vi "Message Log Exited MHLC.vi"(8 "error in (no error)":errorcluster, 10 "Data in":variant, 11 "Debug Server in":refnum<class "Debug Server.lvclass">) -> (0 "error out":errorcluster, 3 "Debug Server out":refnum<class "Debug Server.lvclass">)   [LabVIEW 2017, in "Debug Server.lvclass"]
doc: "A Message Log has exited. Remove it from the array of open Message Logs. Tell TCP Server that the Message Log no longer exists."
uses:
  Debug Server.lvclass
  C:/Program Files (x86)/National Instruments/LabVIEW 2017/vi.lib/addons/_Workers/Library/Classes/Worker/Worker.lvclass
  Debug Server.lvclass/Debug Server.ctl
  Debug Server TCP Server and Client/Workers/DS TCP Server/rqp_Message Log Exited.ctl
  Common VIs/DC_UID.ctl
  <vilib>/Utility/error.llb/Error Cluster From Error Code.vi
  <vilib>/ErrorRing/Error Ring.xnode
  Message Log/Message Log.lvclass
  Debug Server TCP Server and Client/Workers/DS TCP Server/DS TCP Server.lvclass
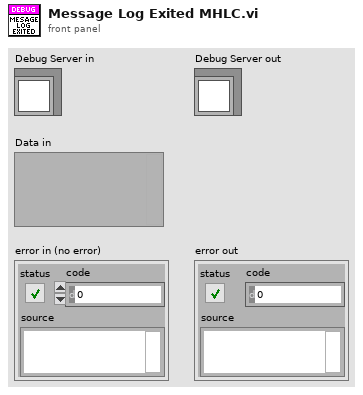
[diagram p1: front panel]
types:
  T1 = typedef "Message Log.lvclass/rsp_Message Log Exited.ctl" = cluster{"Message Log ID":T2}
  T2 = typedef "Message Log ID.ctl" = cluster{"Head Worker ID":string, "IP Address":string}
  T3 = typedef "Debug Server.lvclass/Dynamic Message Log Data.ctl" = cluster{"Message Log":refnum<class "Message Log.lvclass">, "DC_UID":T4, "Message Log ID":T2}
  T4 = typedef "DC_UID.ctl" = string
  T5 = typedef "DS TCP Server.lvlib/DS TCP Server.lvclass/rqp_Message Log Exited.ctl" = cluster{"DC_UID":T4}
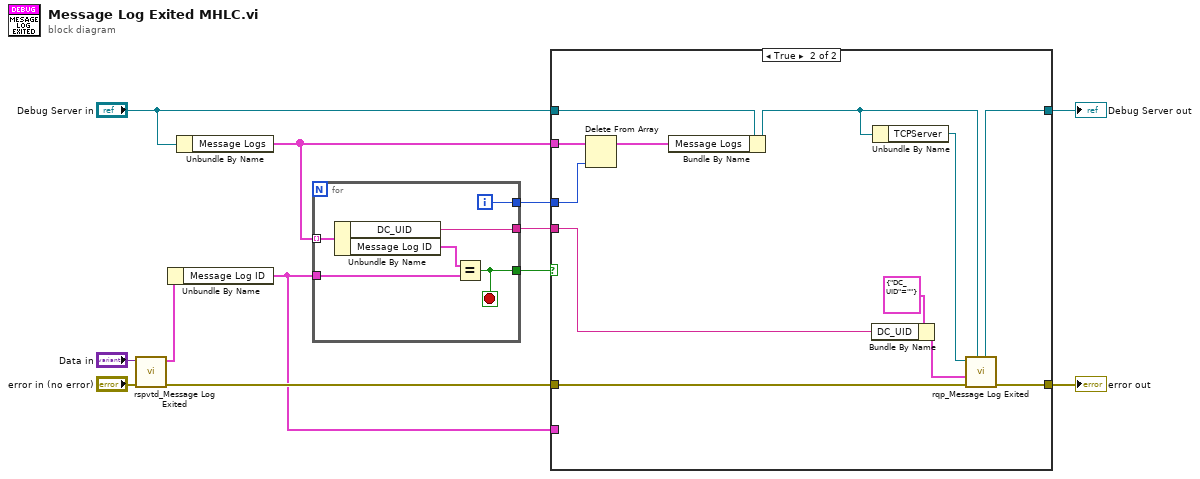
[diagram p0: block diagram]
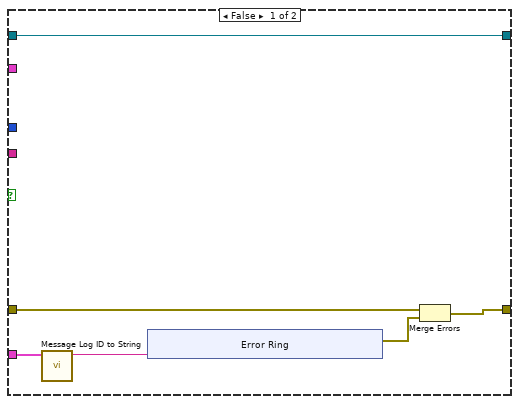
[diagram p2: hidden frame]
diagram:
  n1 = call "rspvtd_Message Log Exited.vi"("error in"="error in (no error)", "Data in"="Data in") -> ("error out"=w9:errorcluster, "Data out"=w6:T1)  [unwired: 8 in]
  n2 = Unbundle By Name(w6) -> ("Message Log ID"=w2:T2)
  n3 = Unbundle By Name("Debug Server in") -> ("Message Logs"=w5:T3[])
  n4 = for {
    tunnel: w5 -> [w18] mode=indexing
    tunnel: [w16] -> w4
    tunnel: [w15] -> w1
    tunnel: w2 -> [w14]
    tunnel: [w13] -> w3
    i -> [w13]
    stop <- w16 stop-if-true
    n5 = Unbundle By Name(w18) -> ("DC_UID"=w15:T4, "Message Log ID"=w17:T2)
    n6 = Equal?(x=w17, y=w14) -> (x = y?=w16:bool)
  }
  n7 = case shown="True" w4 {
    tunnel: [w24 w42] -> w12
    tunnel: [w22 w41] -> w11
    tunnel: w9 -> [w23 w40]
    tunnel: "Debug Server in" -> [w24 w39]
    tunnel: w5 -> [_ w37]
    tunnel: w3 -> [_ w35]
    tunnel: w2 -> [w20 _]
    tunnel: w1 -> [_ w32]
    frame False {
      n8 = call "Message Log ID to String.vi"("Message Log ID"=w20) -> ("Message Log ID String"=w19:string)  [unwired: 10 in]
      n9 = xnode "Error Ring"("parameter 0"=w19) -> ("error out"=w21:errorcluster)
      n10 = Merge Errors(w23, w21) -> (w22:errorcluster)
    }
    frame True {
      n11 = Delete From Array(array=w37, index=w35) -> (array with subset deleted=w36:T3[])  [unwired: 1 in, 1 out]
      n12 = Bundle By Name(cluster=w39, "Message Logs"=w36) -> (w38:refnum<class "Debug Server.lvclass">)
      n13 = Bundle By Name(cluster=T5 {"DC_UID"=""} ("Data in"), "DC_UID"=w32) -> (w33:T5)
      n14 = Unbundle By Name(w38) -> ("TCPServer"=w43:refnum<class "DS TCP Server.lvclass">)
      n15 = call "rqp_Message Log Exited.vi"("Caller in"=w38, "error in"=w40, "Data in"=w33, "DS TCP Server in"=w43) -> ("error out"=w41:errorcluster, "dup Caller out"=w42:refnum<class "Debug Server.lvclass">)  [unwired: 5 in, 1 out]
    }
  }
  "Debug Server out" <- w12
  "error out" <- w11
